vi "N6700_OUTPUT_COUPLE.vi"(0 "VISA session":refnum<visa-resource-name>="TCPIP0::169.254.70.130::inst0::INSTR", 2 "RO(T)":bool, 11 "error in (no error)":errorcluster, 13 "Enable Couple (t)":bool, 14 "Use OPC(T)":bool) -> (4 "dup VISA session":refnum<visa-resource-name>, 8 "read_out_coup_on(t)":bool, 15 "error out":errorcluster)   [LabVIEW 2018]
doc: "This VI configures the DC voltage level the power supply attempts to generate.\n\nVer 3.0.0 supports the E36xx Model and The 6634B based on the GPIB address of idtATE [10-12]"
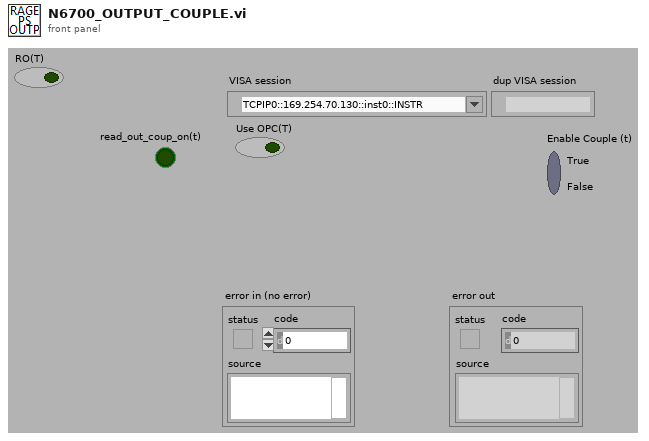
[diagram p1: front panel]
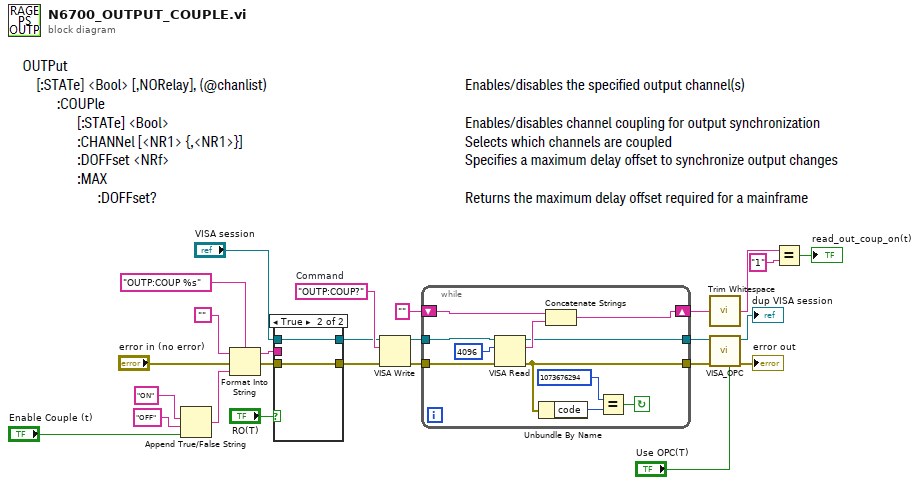
[diagram p0: block diagram]
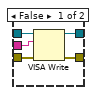
[diagram p2: hidden frame]
diagram:
  w12 = "OUTP:COUP?"  # Command
  n1 = Append True/False String(1:"Enable Couple (t)", 2:"OFF", 3:"ON") -> (0:w19:string)  [unwired: 1 in]
  n2 = Format Into String(format string="OUTP:COUP %s", initial string="", error in="error in (no error)", w19) -> (resulting string=w11:string, error out=w10:errorcluster)
  n3 = case shown="True" "RO(T)" {
    tunnel: w11 -> [w31 _]
    tunnel: [w30 w32] -> w8
    tunnel: w10 -> [w29 w33]
    tunnel: [w28 w33] -> w9
    tunnel: "VISA session" -> [w27 w32]
    frame False {
      n4 = VISA Write(VISA resource name=w27, write buffer=w31, error in (no error)=w29) -> (VISA resource name out=w30:refnum<visa-resource-name>, error out=w28:errorcluster)  [unwired: 1 out]
    }
    frame True {
    }
  }
  n5 = VISA Write(VISA resource name=w8, write buffer=w12, error in (no error)=w9) -> (VISA resource name out=w15:refnum<visa-resource-name>, error out=w14:errorcluster)  [unwired: 1 out]
  n6 = while {
    tunnel: w15 -> [w41]
    shift-right: [w35] -> w4
    shift-left: "" -> [w40]
    tunnel: w14 -> [w38]
    tunnel: [w37] -> w21
    tunnel: [w34] -> w22
    stop <- w36 continue-if-true
    n7 = VISA Read(VISA resource name=w41, byte count=u32 4096 ("byte count (0)"), error in (no error)=w38) -> (VISA resource name out=w34:refnum<visa-resource-name>, read buffer=w39:string, error out=w37:errorcluster)  [unwired: 1 out]
    n8 = Unbundle By Name(w37) -> ("code"=w43:i32)
    n9 = Concatenate Strings(w40, w39) -> (w35:string)
    n10 = Equal?(x=1073676294, y=w43) -> (x = y?=w36:bool)
  }
  n11 = call <vilib>:"Trim Whitespace.vi"("string"=w4) -> ("trimmed string"=w1:string)  [unwired: 1 in]
  n12 = call "VISA_OPC.vi"("OPC(T)"="Use OPC(T)", "error in"=w21, "Session In"=w22) -> ("error out"=→"error out":errorcluster, "Session Out"=→"dup VISA session":refnum<visa-resource-name>)  [unwired: 6 in, 1 out]
  n13 = Equal?(x=w1, y="1") -> (x = y?=→"read_out_coup_on(t)":bool)
